vi "LVDimInterface.application example serv command.vi"() -> ()   [LabVIEW 2015, in "LVDimInterface.lvlib"]
doc: "This VI implements a DIM server, that receives commands via a message queue."
uses:
  LVDimInterface.lvlib
  LVDimInterface.dis_add_command_queue.vi
panel:
  out "error out":errorcluster
  out "data":i32=-1
  out "callBackID":i32=-1
  in  "serverName":string="test27"
  out "received commands":i32=-1
  out "loop counter":i32
  in  "stop":bool
  in  "commandName":string="testCommand"
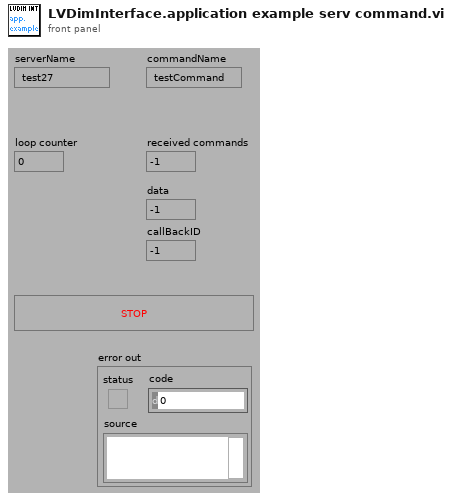
[diagram p1: front panel]
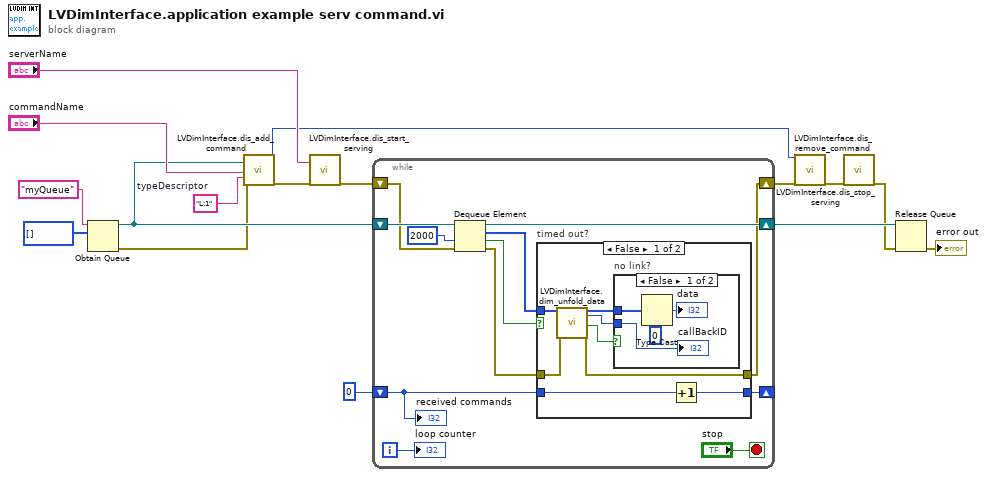
[diagram p0: block diagram]
diagram:
  w6 = "L:1"  # typeDescriptor
  n1 = Obtain Queue(name (unnamed)="myQueue" ("test1"), element data type=i8[] []) -> (queue out=w5:refnum<queue>, error out=w3:errorcluster)  [unwired: 3 in, 1 out]
  n2 = call-poly "LVDimInterface.dis_add_command.vi"("queueRef"=w5, "commandName"="commandName", "typeDescriptor"=w6, "error in (no error)"=w3) -> ("commandID"=w10:i32, "error out"=w12:errorcluster)  [unwired: 14 in]
  n3 = call "LVDimInterface.dis_start_serving.vi"("serverName"="serverName", "error in (no error)"=w12) -> ("error out"=w14:errorcluster)  [unwired: 16 in, 1 out]
  n4 = while {
    shift-right: [w21] -> _
    shift-left: 0 -> [w22]
    shift-right: [w17] -> w8
    shift-left: w14 -> [w18]
    shift-right: [w20] -> w4
    shift-left: w5 -> [w27]
    i -> [w25]
    stop <- "stop" stop-if-true
    n5 = Dequeue Element(queue=w27, timeout in ms (-1)=2000, error in (no error)=w18) -> (queue out=w20:refnum<queue>, element=w24:i8[], timed out?=w23:bool, error out=w19:errorcluster)
    n6 = case "timed out?" shown="False" w23 {
      tunnel: w24 -> [w34 _]
      tunnel: [w35 w42] -> w21
      tunnel: w22 -> [w36 w42]
      tunnel: w19 -> [w30 w41]
      tunnel: [w29 w41] -> w17
      frame False {
        n7 = call "LVDimInterface.dim_unfold_data.vi"("rawData"=w34, "error in (no error)"=w30) -> ("data"=w33:i8[], "callBackID"=w32:i32, "no link"=w31:bool, "error out"=w29:errorcluster)  [unwired: 14 in]
        n8 = case "no link?" shown="False" w31 {
          tunnel: w33 -> [w40 _]
          tunnel: w32 -> [w39 _]
          frame False {
            n9 = Type Cast(type=0, x=w40) -> (*(type *) &x=→"data":i32)
            "callBackID" <- w39
          }
          frame True {
          }
        }
        n10 = Increment(x=w36) -> (x+1=w35:i32)
      }
      frame True {
      }
    }
    "loop counter" <- w25
    "received commands" <- w22
  }
  n11 = call "LVDimInterface.dis_remove_command.vi"("commandID"=w10, "error in (no error)"=w8) -> ("error out"=w9:errorcluster)  [unwired: 17 in]
  n12 = call "LVDimInterface.dis_stop_serving.vi"("error in (no error)"=w9) -> ("error out"=w2:errorcluster)  [unwired: 18 in]
  n13 = Release Queue(queue=w4, error in (no error)=w2) -> (error out=→"error out":errorcluster)  [unwired: 1 in, 2 out]
